vi "test Set Endpoint Configuration Updates Possible Connections.vi"(8 "error in (no error)":errorcluster, 11 "TestCase in":refnum<class "SLSC Switch Scripting Unit Tests.lvclass">) -> (0 "error out":errorcluster, 3 "TestCase out":refnum<class "SLSC Switch Scripting Unit Tests.lvclass">)   [LabVIEW 2019, in "SLSC Switch Scripting Unit Tests.lvclass"]
uses:
  SLSC Switch Scripting Unit Tests.lvclass
  Properties/SLSC Switch All Properties.ctl
  Shared/Routing and Faulting Hardware API/Types/Possible Connections for Endpoint.ctl
  Shared/Endpoint Configuration Enum.ctl
  SLSC Switch Scripting Unit Tests.lvclass/SLSC Switch Scripting Unit Tests.ctl
  Custom Device/Find All SLSC Switch Custom Devices.vi
  <vilib>/addons/_JKI Toolkits/VI Tester/TestCase.llb/TestCase.lvclass
  SLSC Switch Scripting.lvlib
  Shared/Routing and Faulting Hardware API/Routing and Faulting Hardware API.lvlib
  Shared/SLSC Switch Shared.lvlib
  C:/Program Files (x86)/National Instruments/LabVIEW 2019/vi.lib/addons/_JKI Toolkits/VI Tester/TestCase.llb/TestCase.lvclass
panel:
  in  "Save?":bool
  out "Output Filename":string
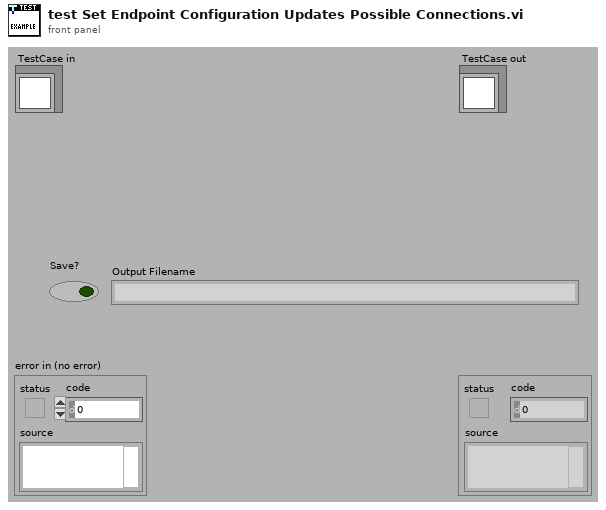
[diagram p1: front panel]
types:
  T1 = typedef "SLSC Switch Shared.lvlib/Endpoint Configuration Enum.ctl" = enum16{"Load", "Source", "Configuration"}
  T2 = typedef "Routing and Faulting Hardware API.lvlib/Possible Connections for Endpoint.ctl" = cluster{"Source":string, "Destinations":string[]}
  T3 = typedef "SLSC Switch Scripting.lvlib/SLSC Switch All Properties.ctl" = cluster{"Product Name":string, "Topology":string, "Switches JSON":string, "Description":string, "Reservation Group":string}
  T4 = typedef "Custom Device API.lvlib/Custom Device Item Ref.ctl" = u64
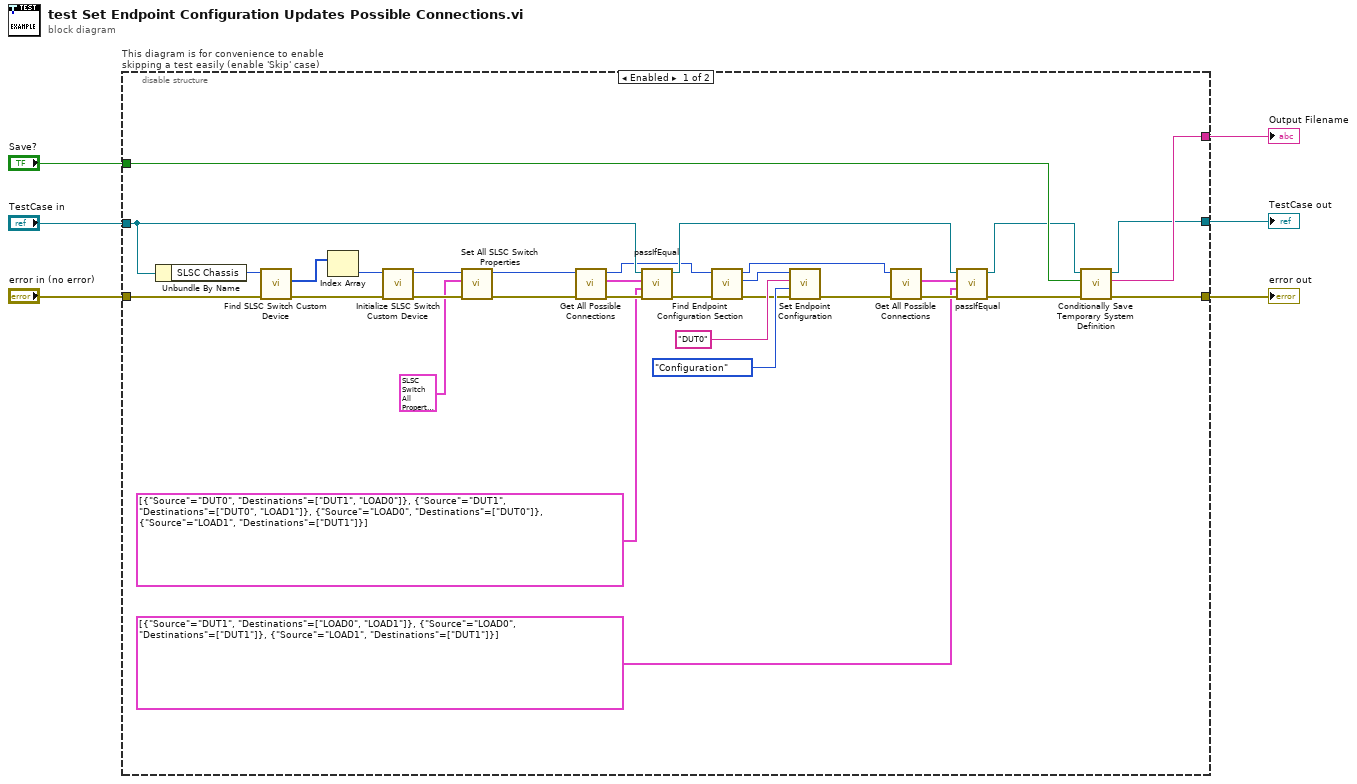
[diagram p0: block diagram]
diagram:
  n1 = disable-structure "This diagram is for convenience to enable skipping a test easily (enable 'Skip' case)" shown="Enabled" {
    disable-tunnel: "TestCase in" -> [w23 w42]
    disable-tunnel: [w36 w40] -> w3
    disable-tunnel: [w37 w41] -> w5
    disable-tunnel: "error in (no error)" -> [w30 w39]
    disable-tunnel: [w38 _] -> w2
    disable-tunnel: "Save?" -> [w35 _]
    frame Enabled {
      n2 = Unbundle By Name(w23) -> ("SLSC Chassis"=w31:u64)
      n3 = call-poly "Find SLSC Switch Custom Device.vi"("error in"=w30, "slsc chassis in"=w31) -> ("error out"=w33:errorcluster, "slsc switch custom devices"=w34:T4[])  [unwired: 7 in, 1 out]
      n4 = Index Array(array=w34) -> (element=w32:T4)  [unwired: 1 in]
      n5 = call "Initialize SLSC Switch Custom Device.vi"("error in"=w33, "slsc switch custom device in"=w32) -> ("error out"=w28:errorcluster, "slsc switch custom device out"=w29:T4)  [unwired: 7 in, 1 out]
      n6 = call "Set All SLSC Switch Properties.vi"("error in"=w28, "properties"=T3 {"Product Name"="Fake Device", "Topology"="SimpleTopology", "Switches JSON"="{\n   \"switchesSpecVersion\": 1,\n   \"relays\": [\n      {\n         \"name\": \"DUT0_LOAD0\",\n         \"actions\": [\n            {\n               \"type\": \"property\",\n               \"resource\": \"Foo\",\n               \"value\": \"Vendor.DUT0_LOAD0\"\n            },\n            {\n               \"type\": \"command\",\n               \"resource\": \"Foo\",\n               \"value\": \"Vendor.Update\"\n            }\n         ]\n      },\n      {\n         \"name\": \"DUT1_LOAD1\",\n         \"actions\": [\n            {\n               \"type\": \"property\",\n               \"resource\": \"Foo\",\n               \"value\": \"Vendor.DUT1_LOAD1\"\n            },\n            {\n               \"type\": \"command\",\n               \"resource\": \"Foo\",\n               \"value\": \"Vendor.Update\"\n            }\n         ]\n      },\n      {\n         \"name\": \"DUT0_DUT1\",\n         \"actions\": [\n            {\n               \"type\": \"property\",\n               \"resource\": \"Foo\",\n               \"value\": \"Vendor.DUT0_DUT1\"\n            },\n            {\n               \"type\": \"command\",\n               \"resource\": \"Foo\",\n               \"value\": \"Vendor.Update\"\n            }\n         ]\n      }\n   ],\n   \"topologies\": [\n      {\n         \"name\": \"SimpleTopology\",\n         \"initialState\": {\n            \"open\": [\n               \"DUT0_LOAD0\",\n               \"DUT1_LOAD1\",\n               \"DUT0_DUT1\"\n            ],\n            \"close\": []\n         },\n         \"channelList\": {\n            \"names\": [\n               \"DUT0\",\n               \"DUT1\",\n               \"LOAD0\",\n               \"LOAD1\"\n            ]\n         },\n         \"connectionList\": [\n            {\n               \"src\": \"DUT0\",\n               \"dest\": \"LOAD0\",\n               \"relays\": [\n                  \"DUT0_LOAD0\"\n               ]\n            },\n            {\n               \"src\": \"DUT1\",\n               \"dest\": \"LOAD1\",\n               \"relays\": [\n                  \"DUT1_LOAD1\"\n               ]\n            },\n            {\n               \"src\": \"DUT0\",\n               \"dest\": \"DUT1\",\n               \"relays\": [\n                  \"DUT0_DUT1\"\n               ]\n            }\n         ]\n      },\n      {\n         \"name\": \"EvenSimplerTopology\",\n         \"initialState\": {\n            \"open\": [\n               \"DUT0_LOAD0\",\n               \"DUT1_LOAD1\"\n            ],\n            \"close\": []\n         },\n         \"channelList\": {\n            \"names\": [\n               \"DUT0\",\n               \"DUT1\",\n               \"LOAD0\",\n               \"LOAD1\"\n            ]\n         },\n         \"connectionList\": [\n            {\n               \"src\": \"DUT0\",\n               \"dest\": \"LOAD0\",\n               \"relays\": [\n                  \"DUT0_LOAD0\"\n               ]\n            },\n            {\n               \"src\": \"DUT1\",\n               \"dest\": \"LOAD1\",\n               \"relays\": [\n                  \"DUT1_LOAD1\"\n               ]\n            }\n         ]\n      }\n   ],\n   \"multiStateRelays\": []\n}", "Description"="", "Reservation Group"=""} ("SLSC Switch All Properties"), "slsc switch custom device in"=w29) -> ("error out"=w26:errorcluster, "slsc switch custom device out"=w25:T4)  [unwired: 7 in]
      n7 = call "Get All Possible Connections.vi"("error in (no error)"=w26, "Hardware Ref in"=w25) -> ("error out"=w24:errorcluster, "Possible Connections"=w20:T2[], "Hardware Ref out"=w9:T4)  [unwired: 6 in, 1 out]
      n8 = call-dynamic "passIfEqual.vi"("error in (no error)"=w24, "y"=T2[] [{"Source"="DUT0", "Destinations"=["DUT1", "LOAD0"]}, {"Source"="DUT1", "Destinations"=["DUT0", "LOAD1"]}, {"Source"="LOAD0", "Destinations"=["DUT0"]}, {"Source"="LOAD1", "Destinations"=["DUT1"]}] ("Possible Connections"), "x"=w20, "TestCase in"=w23) -> ("error out"=w22:errorcluster, "TestCase out"=w16:refnum<class "SLSC Switch Scripting Unit Tests.lvclass">)  [unwired: 6 in]
      n9 = call "Find Endpoint Configuration Section.vi"("error in"=w22, "slsc switch custom device in"=w9) -> ("error out"=w10:errorcluster, "endpoint configuration"=w8:T4, "slsc switch custom device out"=w7:T4)  [unwired: 7 in]
      n10 = call "Set Endpoint Configuration.vi"("error in"=w10, "configuration"=Endpoint_Configuration_Enum."Configuration" ("Configuration Type"), "endpoint"="DUT0" ("Endpoint"), "endpoint configuration in"=w8) -> ("error out"=w17:errorcluster)  [unwired: 6 in, 1 out]
      n11 = call "Get All Possible Connections.vi"("error in (no error)"=w17, "Hardware Ref in"=w7) -> ("error out"=w19:errorcluster, "Possible Connections"=w18:T2[])  [unwired: 6 in, 2 out]
      n12 = call-dynamic "passIfEqual.vi"("error in (no error)"=w19, "y"=T2[] [{"Source"="DUT1", "Destinations"=["LOAD0", "LOAD1"]}, {"Source"="LOAD0", "Destinations"=["DUT1"]}, {"Source"="LOAD1", "Destinations"=["DUT1"]}] ("Possible Connections"), "x"=w18, "TestCase in"=w16) -> ("error out"=w14:errorcluster, "TestCase out"=w15:refnum<class "SLSC Switch Scripting Unit Tests.lvclass">)  [unwired: 6 in]
      n13 = call "Conditionally Save Temporary System Definition.vi"("error in (no error)"=w14, "Save?"=w35, "Test Case"=w15) -> ("error out"=w37:errorcluster, "filename"=w38:string, "Test Case"=w36:refnum<class "SLSC Switch Scripting Unit Tests.lvclass">)  [unwired: 6 in]
    }
    frame Disabled {
      # "skip test result while test is under development"
      n14 = call <vilib>:"skip.vi"("error in (no error)"=w39, "TestCase in"=w42) -> ("error out"=w41:errorcluster, "TestCase out"=w40:refnum<class "SLSC Switch Scripting Unit Tests.lvclass">)  [unwired: 8 in]
    }
  }
  "error out" <- w5
  "TestCase out" <- w3
  "Output Filename" <- w2
